vi "testConvertToKeyValuePairWithJSON.vi"(8 "error in (no error)":errorcluster) -> (0 "error out":errorcluster)   [LabVIEW 2018]
doc: "Test the convertToKeyValuePair.vi with Unflatten from JSON function."
uses:
  src/Utility/keyValuePair/convertToKeyValuePair_double.vi
  src/Utility/keyValuePair/convertToKeyValuePair_integer32bit.vi
  src/Utility/keyValuePair/convertToKeyValuePair_boolean.vi
  src/Utility/keyValuePair/convertToKeyValuePair_string.vi
  src/Utility/keyValuePair/convertToKeyValuePair_1Ddouble.vi
  src/Utility/keyValuePair/convertToKeyValuePair_2Ddouble.vi
  <vilib>/addons/_JKI Toolkits/Caraya/classes/Assert/Assert Equal Value_Variant.vi
  src/Utility/keyValuePair/convertToKeyValuePair_integer64bit.vi
  src/Utility/keyValuePair/convertToKeyValuePair_unsignedInteger32bit.vi
  src/Utility/keyValuePair/convertToKeyValuePair_unsignedInteger64bit.vi
  src/Utility/keyValuePair/convertToKeyValuePair_1Dstring.vi
  <vilib>/addons/_JKI Toolkits/Caraya/classes/Test/Test.lvclass
  <vilib>/addons/_JKI Toolkits/Caraya/classes/Assert/Assert.lvclass
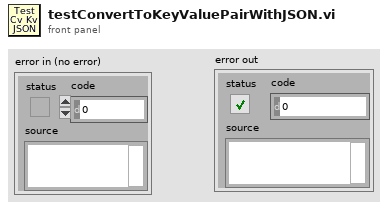
[diagram p1: front panel]
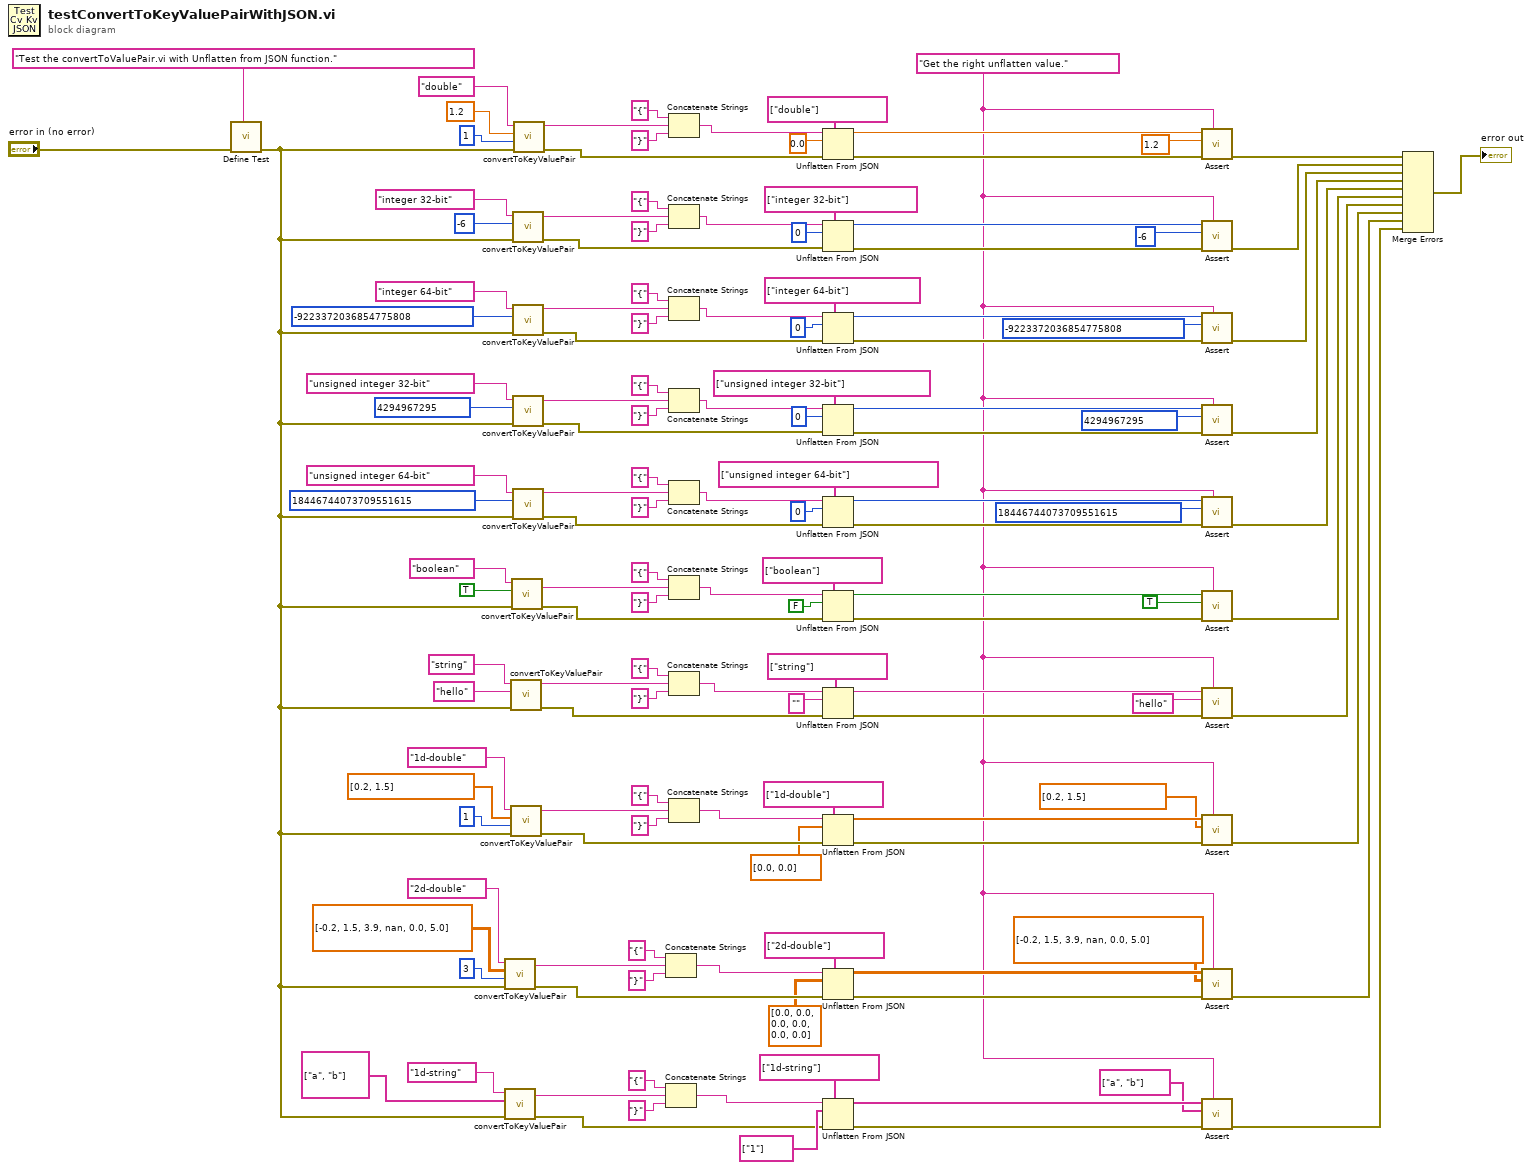
[diagram p0: block diagram]
diagram:
  w5 = "Get the right unflatten value." ("Label")
  n1 = call <vilib>:"Define Test.vi"("error in (no error)"="error in (no error)", "Label (VI Title)"="Test the convertToValuePair.vi with Unflatten from JSON function.") -> ("error out"=w14:errorcluster)  [unwired: 9 in]
  n2 = call-poly "convertToKeyValuePair.vi"("error in (no error)"=w14, "presicion (0)"=u8 3 ("precision (0)"), "value"=dbl[][] [[-0.2, 1.5, 3.9], [nan, 0.0, 5.0]], "name"="2d-double") -> ("error out"=w87:errorcluster, "string converted"=w102:string)  [unwired: 6 in]
  n3 = call-poly "convertToKeyValuePair.vi"("error in (no error)"=w14, "value"=string[] ["a", "b"], "name"="1d-string") -> ("error out"=w6:errorcluster, "string converted"=w10:string)  [unwired: 7 in]
  n4 = call-poly "convertToKeyValuePair.vi"("error in (no error)"=w14, "value"="hello", "name"="string") -> ("error out"=w90:errorcluster, "string converted"=w104:string)  [unwired: 7 in]
  n5 = call-poly "convertToKeyValuePair.vi"("error in (no error)"=w14, "presicion (0)"=u8 1 ("precision (0)"), "value"=dbl[] [0.2, 1.5], "name"="1d-double") -> ("error out"=w89:errorcluster, "string converted"=w103:string)  [unwired: 6 in]
  n6 = call-poly "convertToKeyValuePair.vi"("error in (no error)"=w14, "value"=TRUE, "name"="boolean") -> ("error out"=w93:errorcluster, "string converted"=w105:string)  [unwired: 7 in]
  n7 = call-poly "convertToKeyValuePair.vi"("error in (no error)"=w14, "value"=-6, "name"="integer 32-bit") -> ("error out"=w95:errorcluster, "string converted"=w106:string)  [unwired: 7 in]
  n8 = call-poly "convertToKeyValuePair.vi"("error in (no error)"=w14, "value"=i64 -9223372036854775808, "name"="integer 64-bit") -> ("error out"=w49:errorcluster, "string converted"=w48:string)  [unwired: 7 in]
  n9 = call-poly "convertToKeyValuePair.vi"("error in (no error)"=w14, "value"=u32 4294967295, "name"="unsigned integer 32-bit") -> ("error out"=w25:errorcluster, "string converted"=w23:string)  [unwired: 7 in]
  n10 = call-poly "convertToKeyValuePair.vi"("error in (no error)"=w14, "value"=u64 18446744073709551615, "name"="unsigned integer 64-bit") -> ("error out"=w37:errorcluster, "string converted"=w38:string)  [unwired: 7 in]
  n11 = call-poly "convertToKeyValuePair.vi"("error in (no error)"=w14, "precision (0)"=u8 1, "value"=1.2, "name"="double") -> ("error out"=w96:errorcluster, "string converted"=w133:string)  [unwired: 6 in]
  n12 = Concatenate Strings("{", w102, "}") -> (w97:string)
  n13 = Concatenate Strings("{", w10, "}") -> (w7:string)
  n14 = Concatenate Strings("{", w133, "}") -> (w120:string)
  n15 = Concatenate Strings("{", w106, "}") -> (w101:string)
  n16 = Concatenate Strings("{", w48, "}") -> (w52:string)
  n17 = Concatenate Strings("{", w23, "}") -> (w24:string)
  n18 = Concatenate Strings("{", w38, "}") -> (w34:string)
  n19 = Concatenate Strings("{", w105, "}") -> (w100:string)
  n20 = Concatenate Strings("{", w104, "}") -> (w99:string)
  n21 = Concatenate Strings("{", w103, "}") -> (w98:string)
  n22 = Unflatten From JSON(path=string[] ["double"], JSON string=w120, type and defaults=0.0 ("value"), error in (no error)=w96) -> (value=w84:dbl, error out=w82:errorcluster)  [unwired: 3 in]
  n23 = Unflatten From JSON(path=string[] ["integer 32-bit"], JSON string=w101, type and defaults=0 ("value"), error in (no error)=w95) -> (value=w75:i32, error out=w81:errorcluster)  [unwired: 3 in]
  n24 = Unflatten From JSON(path=string[] ["integer 64-bit"], JSON string=w52, type and defaults=i64 0 ("value"), error in (no error)=w49) -> (value=w45:i64, error out=w47:errorcluster)  [unwired: 3 in]
  n25 = Unflatten From JSON(path=string[] ["unsigned integer 32-bit"], JSON string=w24, type and defaults=u32 0 ("value"), error in (no error)=w25) -> (value=w28:u32, error out=w27:errorcluster)  [unwired: 3 in]
  n26 = Unflatten From JSON(path=string[] ["unsigned integer 64-bit"], JSON string=w34, type and defaults=u64 0 ("value"), error in (no error)=w37) -> (value=w40:u64, error out=w39:errorcluster)  [unwired: 3 in]
  n27 = Unflatten From JSON(path=string[] ["boolean"], JSON string=w100, type and defaults=FALSE ("value"), error in (no error)=w93) -> (value=w72:bool, error out=w80:errorcluster)  [unwired: 3 in]
  n28 = Unflatten From JSON(path=string[] ["string"], JSON string=w99, type and defaults="" ("value"), error in (no error)=w90) -> (value=w71:string, error out=w79:errorcluster)  [unwired: 3 in]
  n29 = Unflatten From JSON(path=string[] ["1d-double"], JSON string=w98, type and defaults=dbl[] [0.0, 0.0] ("value"), error in (no error)=w89) -> (value=w70:dbl[], error out=w78:errorcluster)  [unwired: 3 in]
  n30 = Unflatten From JSON(path=string[] ["2d-double"], JSON string=w97, type and defaults=dbl[][] [[0.0, 0.0, 0.0], [0.0, 0.0, 0.0]] ("value"), error in (no error)=w87) -> (value=w77:dbl[][], error out=w76:errorcluster)  [unwired: 3 in]
  n31 = Unflatten From JSON(path=string[] ["1d-string"], JSON string=w7, type and defaults=string[] ["1"], error in (no error)=w6) -> (value=w4:string[], error out=w3:errorcluster)  [unwired: 3 in]
  n32 = call-poly <vilib>:"Assert.vi"("Label"=w5, "error in (no error)"=w82, "Y"=1.2 ("value"), "X"=w84) -> ("error out"=w61:errorcluster)  [unwired: 7 in]
  n33 = call-poly <vilib>:"Assert.vi"("Label"=w5, "error in (no error)"=w81, "Y"=-6 ("value"), "X"=w75) -> ("error out"=w59:errorcluster)  [unwired: 7 in]
  n34 = call-poly <vilib>:"Assert.vi"("Label"=w5, "error in (no error)"=w47, "Y"=i64 -9223372036854775808 ("value"), "X"=w45) -> ("error out"=w46:errorcluster)  [unwired: 7 in]
  n35 = call-poly <vilib>:"Assert.vi"("Label"=w5, "error in (no error)"=w27, "Y"=u32 4294967295 ("value"), "X"=w28) -> ("error out"=w18:errorcluster)  [unwired: 7 in]
  n36 = call-poly <vilib>:"Assert.vi"("Label"=w5, "error in (no error)"=w39, "Y"=u64 18446744073709551615 ("value"), "X"=w40) -> ("error out"=w16:errorcluster)  [unwired: 7 in]
  n37 = call-poly <vilib>:"Assert.vi"("Label"=w5, "error in (no error)"=w80, "Y"=TRUE ("value"), "X"=w72) -> ("error out"=w17:errorcluster)  [unwired: 7 in]
  n38 = call-poly <vilib>:"Assert.vi"("Label"=w5, "error in (no error)"=w79, "Y"="hello" ("value"), "X"=w71) -> ("error out"=w58:errorcluster)  [unwired: 7 in]
  n39 = call-poly <vilib>:"Assert.vi"("Label"=w5, "error in (no error)"=w78, "Y"=dbl[] [0.2, 1.5] ("value"), "X"=w70) -> ("error out"=w57:errorcluster)  [unwired: 7 in]
  n40 = call-poly <vilib>:"Assert.vi"("Label"=w5, "error in (no error)"=w76, "Y"=dbl[][] [[-0.2, 1.5, 3.9], [nan, 0.0, 5.0]] ("value"), "X"=w77) -> ("error out"=w56:errorcluster)  [unwired: 7 in]
  n41 = call-poly <vilib>:"Assert.vi"("Label"=w5, "error in (no error)"=w3, "Y"=string[] ["a", "b"], "X"=w4) -> ("error out"=w1:errorcluster)  [unwired: 7 in]
  n42 = Merge Errors(w61, w59, w46, w18, w16, w17, w58, w57, w56, w1) -> (→"error out":errorcluster)
